vi "derivative_toString.vi"(11 "derivative":T1={"derivative"="derivative", "Interval"=2.0, "Interval Units"=enum."Points", "Type"=enum."dy/dx vs x"}) -> (3 "concatenated string":string)   [LabVIEW 2016]
panel:
  out "error out":errorcluster
  in  "error in":errorcluster
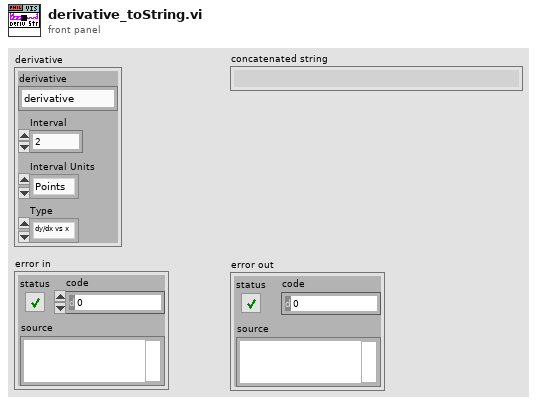
[diagram p1: front panel]
types:
  T1 = cluster{"derivative":string, "Interval":dbl, "Interval Units":enum16{"Points", "Data"}, "Type":enum16{"dy/dx vs x", "dx/dy vs y"}}
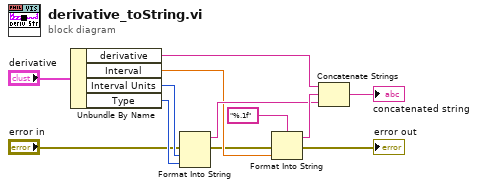
[diagram p0: block diagram]
diagram:
  n1 = Unbundle By Name("derivative") -> ("derivative"=w10:string, "Interval"=w4:dbl, "Interval Units"=w11:enum16{"Points", "Data"}, "Type"=w7:enum16{"dy/dx vs x", "dx/dy vs y"})
  n2 = Format Into String(error in="error in", w11, w7) -> (resulting string=w8:string, error out=w2:errorcluster)  [unwired: 2 in]
  n3 = Format Into String(format string="%.1f", error in=w2, w4) -> (resulting string=w9:string, error out=→"error out":errorcluster)  [unwired: 1 in]
  n4 = Concatenate Strings(w10, w9, w8) -> (→"concatenated string":string)
